vi "close shutter.vi"(8 "error in (no error)":errorcluster, 11 "Murmex in":refnum<class "Murmex.lvclass">) -> (0 "error out":errorcluster, 3 "Murmex out":refnum<class "Murmex.lvclass">)   [LabVIEW 2012]
uses:
  <vilib>/Distrio/Murmex/Murmex/Murmex.lvclass
  <vilib>/Distrio/Murmex/GenericMessage/GenericMessage.lvclass
  <vilib>/Distrio/Murmex/StopMessage/StopMessage.lvclass
  <vilib>/Distrio/Murmex/Message/Add or replace parameter.vi
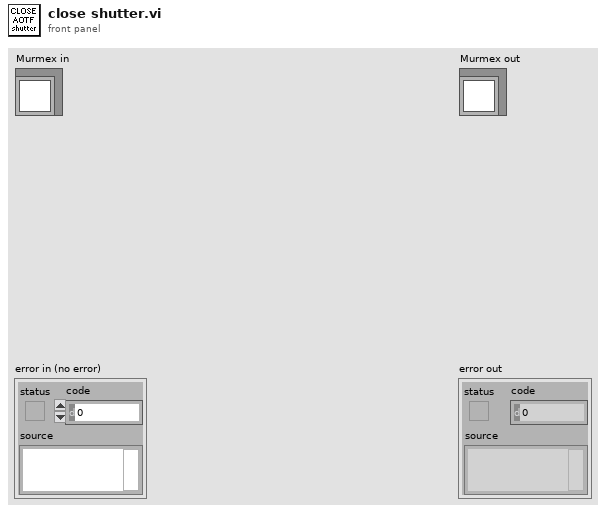
[diagram p1: front panel]
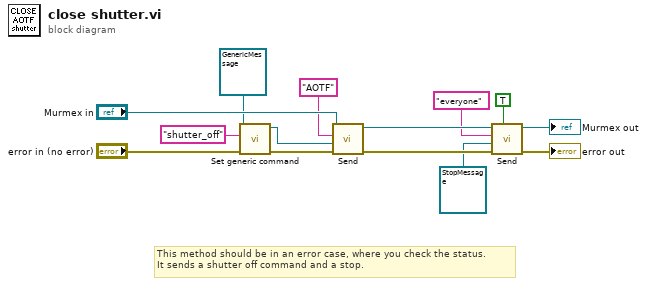
[diagram p0: block diagram]
diagram:
  # "This method should be in an error case, where you check the status.\nIt sends a shutter off command and a stop."
  n1 = call <vilib>:"Set generic command.vi"("error in (no error)"="error in (no error)", "generic command"="shutter_off", "GenericMessage in"=refnum<class "GenericMessage.lvclass"> refnum ("Murmex.lvlib:GenericMessage")) -> ("error out"=w9:errorcluster, "GenericMessage out"=w8:refnum<class "GenericMessage.lvclass">)  [unwired: 7 in]
  n2 = call <vilib>:"Send.vi"("error in (no error)"=w9, "Message"=w8, "recipient"="AOTF", "Murmex in"="Murmex in") -> ("error out"=w4:errorcluster, "Murmex out"=w5:refnum<class "Murmex.lvclass">)  [unwired: 6 in]
  n3 = call <vilib>:"Send.vi"("broadcast? (F)"=TRUE, "error in (no error)"=w4, "Message"=refnum<class "StopMessage.lvclass"> refnum ("Message in"), "recipient"="everyone", "Murmex in"=w5) -> ("error out"=→"error out":errorcluster, "Murmex out"=→"Murmex out":refnum<class "Murmex.lvclass">)  [unwired: 5 in]
